vi "Wait With Error.vi"(7 "milliseconds to wait":u32, 8 "error in (no error)":errorcluster) -> (0 "error out":errorcluster)   [LabVIEW 2018, in "STEPkgDriver_LINC.lvlib"]
doc: "Allows the \"Wait (ms)\" function to be placed between LabVIEW calls that use error cluster error handling and I32 handles. It is functionally equivalent to the \"Wait (ms)\" function. This VI will not wait if there is an incoming error."
uses:
  STEPkgDriver_LINC.lvlib
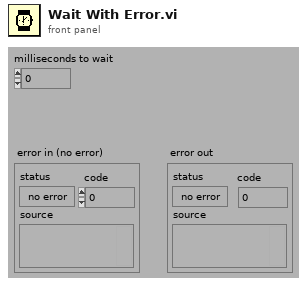
[diagram p1: front panel]
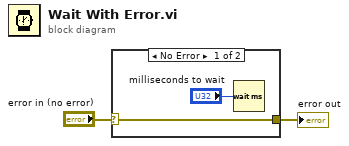
[diagram p0: block diagram]
diagram:
  n1 = case shown="No Error" "error in (no error)" {
    selector: "error in (no error)" -> [w3 w5]
    tunnel: [w3 w5] -> w2
    frame No Error {
      n2 = Wait (ms)(milliseconds to wait="milliseconds to wait") -> ()  [unwired: 1 out]
    }
    frame Error {
    }
  }
  "error out" <- w2
